vi "Circus Launcher.vi"(6 "Launch Local?":bool, 8 "error in (no error)":errorcluster) -> (0 "error out":errorcluster)   [LabVIEW 2020]
uses:
  TALOS/TALOS_PPL.lvlibp
panel:
  # "Launcher of the Circus LabVIEW Code Project (just calling the one in the TALOS PPL)"
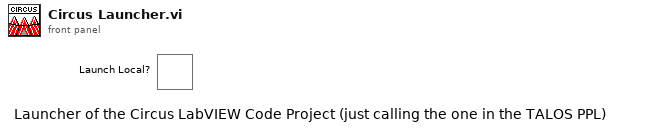
[diagram p1: front panel]
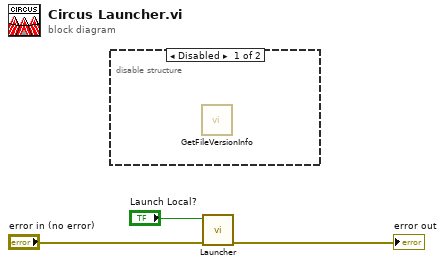
[diagram p0: block diagram]
diagram:
  n1 = disable-structure shown="Disabled" {
    frame Disabled {
      n2 = call <vilib>:"GetFileVersionInfo.vi"() -> ()  [unwired: 10 in, 2 out]
    }
    frame Enabled {
    }
  }
  n3 = call "Launcher.vi"("error in (no error)"="error in (no error)", "Launch Local?"="Launch Local?") -> ("error out"=→"error out":errorcluster)  [unwired: 9 in]
